vi "check if plot is empty.vi"(8 "error in":errorcluster, 11 "App Data in":T1) -> (0 "error out":errorcluster, 2 "record/overwrite?":bool, 3 "App Data out":T1)   [LabVIEW 2014]
uses:
  Controls/App Data.ctl
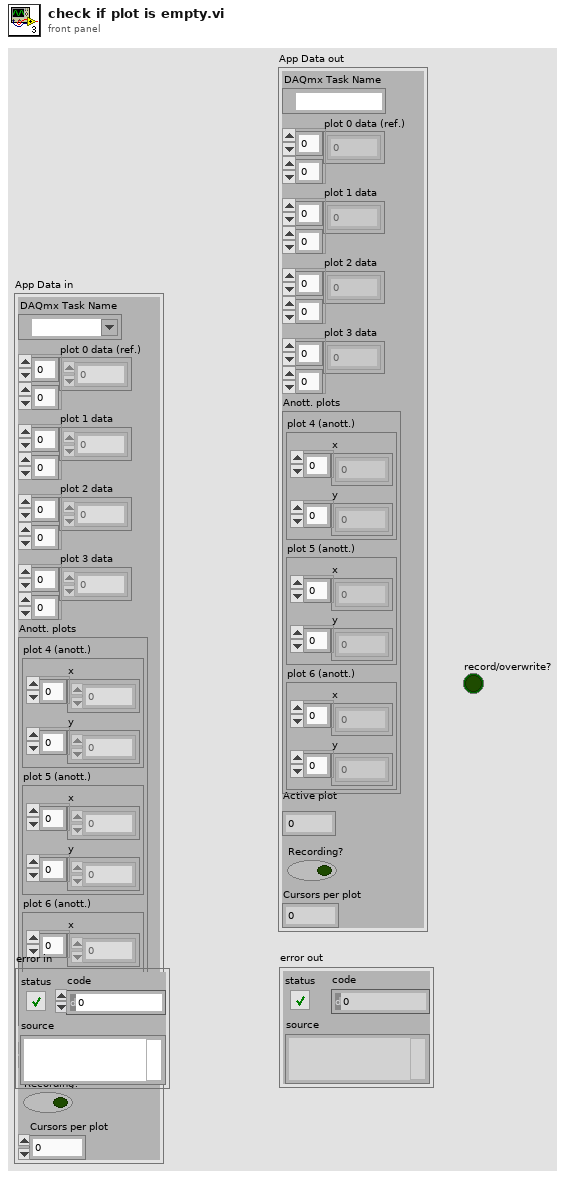
[diagram p1: front panel]
types:
  T1 = typedef "App Data.ctl" = cluster{"DAQmx Task Name":refnum<k21>, "plot 0 data (ref.)":dbl[][], "plot 1 data":dbl[][], "plot 2 data":dbl[][], "plot 3 data":dbl[][], "Anott. plots":cluster{"plot 4 (anott.)":cluster{"x":dbl[], "y":dbl[]}, "plot 5 (anott.)":cluster{"x":dbl[], "y":dbl[]}, "plot 6 (anott.)":cluster{"x":dbl[], "y":dbl[]}}, "Active plot":u32, "Recording?":bool, "Cursors per plot":i32}
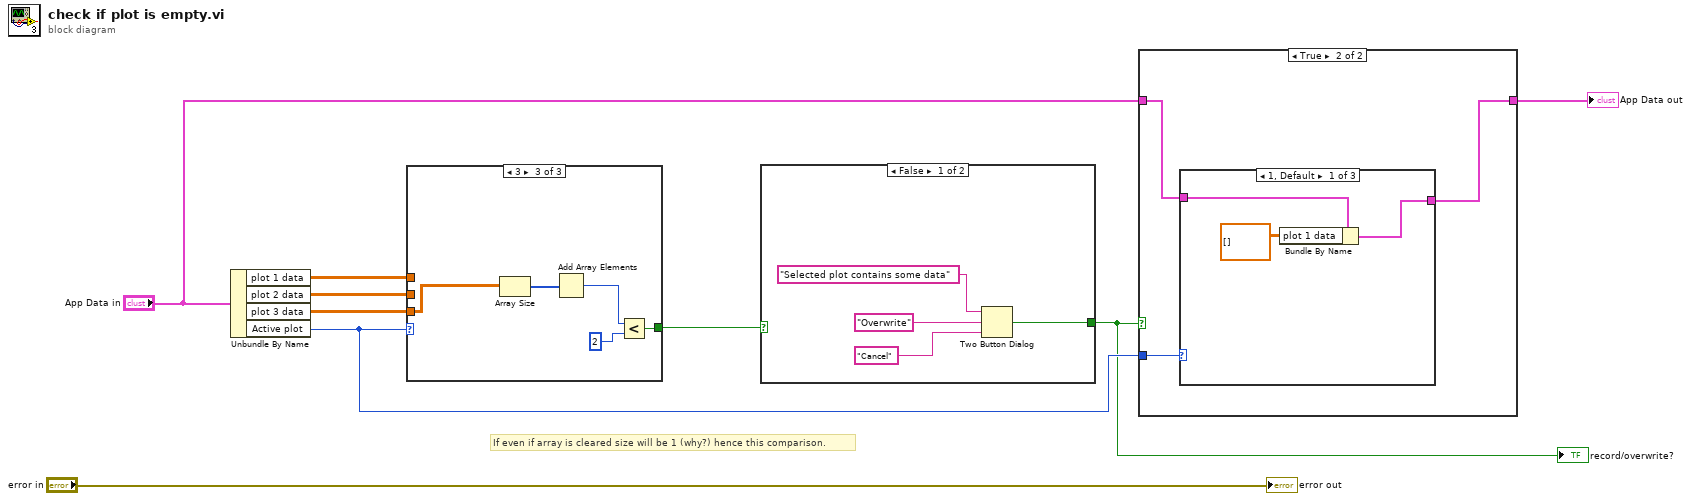
[diagram p0: block diagram]
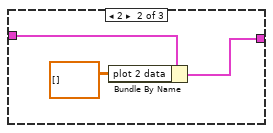
[diagram p3: hidden frame]
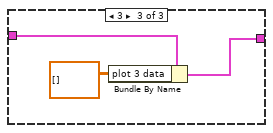
[diagram p4: hidden frame]
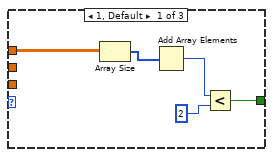
[diagram p6: hidden frame]
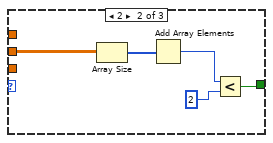
[diagram p7: hidden frame]
diagram:
  # "If even if array is cleared size will be 1 (why?) hence this comparison."
  n1 = Unbundle By Name("App Data in") -> ("plot 1 data"=w9:dbl[][], "plot 2 data"=w8:dbl[][], "plot 3 data"=w7:dbl[][], "Active plot"=w4:u32)
  n2 = case shown="3" w4 {
    tunnel: w9 -> [w14 _ _]
    tunnel: w8 -> [_ w18 _]
    tunnel: w7 -> [_ _ w23]
    tunnel: [w10 w16 w21] -> w6
    frame 1, Default {
      n3 = Array Size(array=w14) -> (size(s)=w13:i32[])
      n4 = Add Array Elements(numeric array=w13) -> (sum=w12:i32)
      n5 = Less?(x=w12, y=2) -> (x < y?=w10:bool)
    }
    frame 2 {
      n6 = Array Size(array=w18) -> (size(s)=w19:i32[])
      n7 = Add Array Elements(numeric array=w19) -> (sum=w15:i32)
      n8 = Less?(x=w15, y=2) -> (x < y?=w16:bool)
    }
    frame 3 {
      n9 = Array Size(array=w23) -> (size(s)=w24:i32[])
      n10 = Add Array Elements(numeric array=w24) -> (sum=w20:i32)
      n11 = Less?(x=w20, y=2) -> (x < y?=w21:bool)
    }
  }
  n12 = case shown="False" w6 {
    selector: w6 -> [_ w29]
    tunnel: [w25 w29] -> w3
    frame False {
      n13 = Two Button Dialog(message="Selected plot contains some data", 1:"Cancel" ("F button name (\"Cancel\")"), 2:"Overwrite" ("T button name (\"OK\")")) -> (T button?=w25:bool)
    }
    frame True {
    }
  }
  "record/overwrite?" <- w3
  n14 = case shown="True" w3 {
    tunnel: w4 -> [_ w33]
    tunnel: "App Data in" -> [w30 w32]
    tunnel: [w30 w31] -> w1
    frame False {
    }
    frame True {
      n15 = case shown="1, Default" w33 {
        tunnel: w32 -> [w36 w39 w42]
        tunnel: [w34 w37 w40] -> w31
        frame 1, Default {
          n16 = Bundle By Name(cluster=w36, "plot 1 data"=dbl[][] []) -> (w34:T1)
        }
        frame 2 {
          n17 = Bundle By Name(cluster=w39, "plot 2 data"=dbl[][] [] ("plot 1 data")) -> (w37:T1)
        }
        frame 3 {
          n18 = Bundle By Name(cluster=w42, "plot 3 data"=dbl[][] [] ("plot 1 data")) -> (w40:T1)
        }
      }
    }
  }
  "App Data out" <- w1
  "error out" <- "error in"
